vi "PmGetSpeeds.vi"(8 "error in (no error)":errorcluster, 11 "reference in":refnum<k24>) -> (0 "error out":errorcluster, 2 "ScanLineTimeUs":dbl, 3 "reference out":refnum<k24>)   [LabVIEW 2022 SP3, in "Photometrics Camera.lvlib"]
uses:
  Photometrics Camera.lvlib
  C:/FlashGordon/Development/dll/PVCamNET.dll
  dll/PVCamNET.dll
panel:
  out "FF Readout (ms)":dbl
  out "Current":string
  out "Speed Names":string[](array[string])
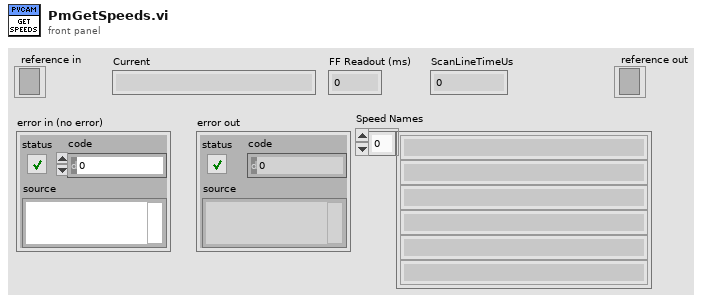
[diagram p1: front panel]
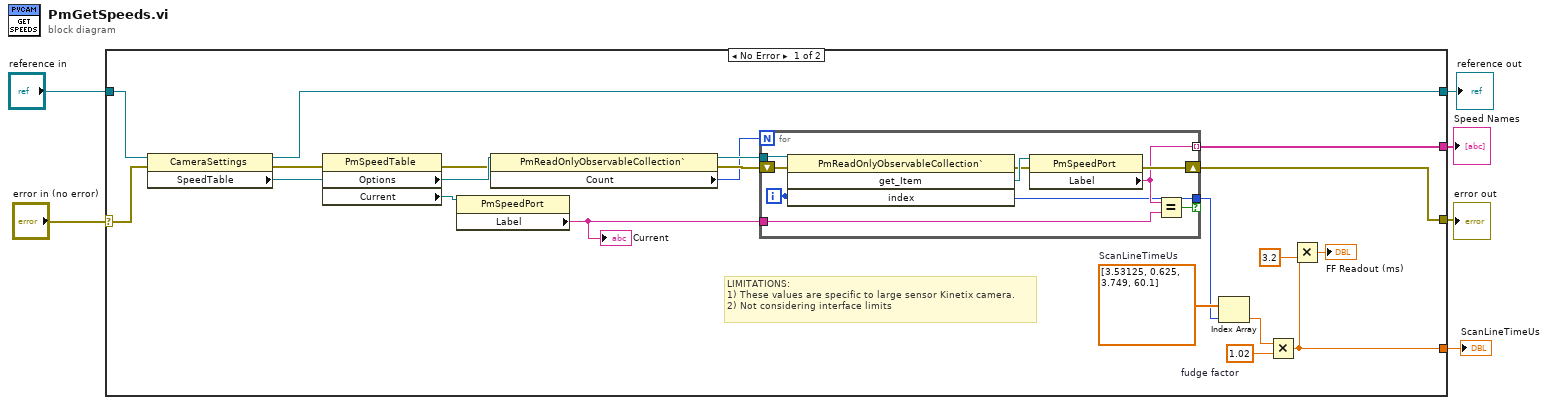
[diagram p0: block diagram]
diagram:
  n1 = case shown="No Error" "error in (no error)" {
    selector: "error in (no error)" -> [w19 w38]
    tunnel: [w27 w38] -> w5
    tunnel: [w26 _] -> w4
    tunnel: "reference in" -> [w17 w37]
    tunnel: [w15 w37] -> w2
    tunnel: [w12 _] -> w1
    frame No Error {
      w7 = 1.02  # fudge factor
      w14 = dbl[] [3.53125, 0.625, 3.749, 60.1]  # ScanLineTimeUs
      # "LIMITATIONS:\n1) These values are specific to large sensor Kinetix camera. \n2) Not considering interface limits"
      n2 = property class="CameraSettings"(reference=w17, error in=w19) -> (reference out=w15:refnum<k24>, error out=w20:errorcluster, "SpeedTable"=w18:refnum<k24>)
      n3 = property class="PmSpeedTable"(reference=w18, error in=w20) -> (error out=w24:errorcluster, "Options"=w25:refnum<k24>, "Current"=w16:refnum<k24>)  [unwired: 1 out]
      n4 = property class="PmSpeedPort"(reference=w16) -> ("Label"=w9:string)  [unwired: 1 in, 2 out]
      "Current" <- w9
      n5 = property class="PmReadOnlyObservableCollection`"(reference=w25, error in=w24) -> (reference out=w22:refnum<k24>, error out=w23:errorcluster, "Count"=w21:i32)
      n6 = for {
        N: w21 -> [_]
        tunnel: [w31] -> w26 mode=indexing
        shift-right: [w32] -> w27
        shift-left: w23 -> [w36]
        tunnel: w22 -> [w35]
        tunnel: w9 -> [w30]
        tunnel: [w29] -> w8 if=w28
        i -> [w29]
        n7 = invoke class="PmReadOnlyObservableCollection`" method="get_Item"(reference=w35, error in=w36, "index"=w29) -> (error out=w33:errorcluster, "get_Item"=w34:refnum<k24>)  [unwired: 1 in, 2 out]
        n8 = property class="PmSpeedPort"(reference=w34, error in=w33) -> (error out=w32:errorcluster, "Label"=w31:string)  [unwired: 1 out]
        n9 = Equal?(x=w31, y=w30) -> (x = y?=w28:bool)
      }
      n10 = Index Array(array=w14, index=w8) -> (element=w13:dbl)
      n11 = Multiply(x=w13, y=w7) -> (x*y=w12:dbl)
      n12 = Multiply(x=w12, y=3.2) -> (x*y=→"FF Readout (ms)":dbl)
    }
    frame Error {
    }
  }
  "error out" <- w5
  "Speed Names" <- w4
  "reference out" <- w2
  "ScanLineTimeUs" <- w1
